vi "Application Error Class Constructor.vi"(0 "Application Error in":refnum<class "Application Error.lvclass">, 1 "Error Scope":string, 2 "Error Name":string, 5 "Error Source":string, 7 "Log Error?":bool, 9 "Call Chain":string[](array[string]), 11 "error in (no error)":errorcluster, 12 "Error Message":string, 13 "Time Stamp":timestamp) -> (15 "error out":errorcluster)   [LabVIEW 2016, in "Stream Error.lvlib" / "Application Error.lvclass"]
doc: "--\nCopyright © 2017 Composed SystemsI All rights reserved.\n\nAuthor: Jon McBee <jon.mcbee@composed.io>\n\nThis library is provided \"AS IS\" ,WITHOUT WARRANTIES OR\nCONDITIONS OF ANY KIND, either express or implied.\n\nComposed Systems -- composed.io\n\nStream 0.0.1.1\nJon McBee - Composed Systems\nCopyright (c) 2017, Composed Systems"
uses:
  <userlib>/Composed Systems/Stream/Error/Classes/Application Error/Application Error.lvclass
  C:/Program Files (x86)/National Instruments/LabVIEW 2016/user.lib/Composed Systems/Stream/Error/Classes/Error Interface/Error Interface.lvclass
  <userlib>/Composed Systems/Stream/Error/Classes/Error Interface/Error Interface.lvclass/Error Interface.ctl
  <userlib>/Composed Systems/Stream/Log/Application Log/Log Level.ctl
  <userlib>/Composed Systems/Stream/Error/Classes/Error Interface/Error Interface.lvclass
  <userlib>/Composed Systems/Stream/Log/Global Application Log/Global Application Log.lvclass
  <userlib>/Composed Systems/Stream/Log/Application Log/Application Log.lvclass
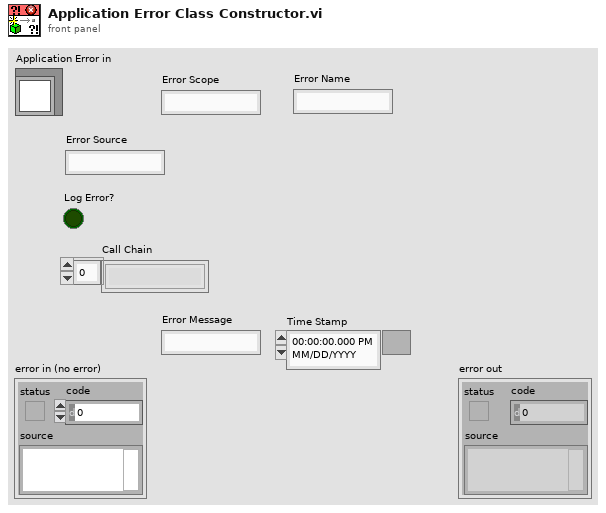
[diagram p1: front panel]
types:
  T1 = typedef "Stream Log.lvlib/Application Log.lvclass/Log Level.ctl" = enum16{"Imperative", "Major", "Minor", "Debug", "Off"}
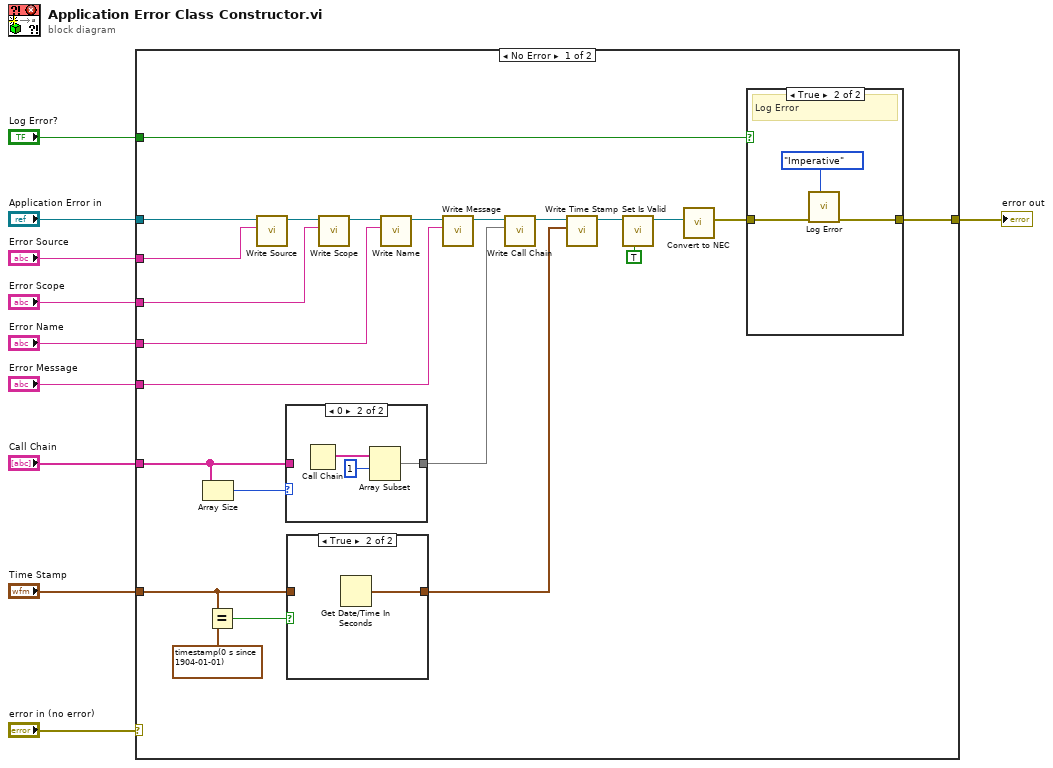
[diagram p0: block diagram]
diagram:
  n1 = case shown="No Error" "error in (no error)" {
    selector: "error in (no error)" -> [_ w44]
    tunnel: "Log Error?" -> [w14 _]
    tunnel: "Time Stamp" -> [w31 _]
    tunnel: "Call Chain" -> [w29 _]
    tunnel: "Error Source" -> [w28 _]
    tunnel: "Error Scope" -> [w27 _]
    tunnel: "Error Name" -> [w21 _]
    tunnel: "Error Message" -> [w20 _]
    tunnel: [w12 w44] -> w1
    tunnel: "Application Error in" -> [w11 _]
    frame No Error {
      n2 = Array Size(array=w29) -> (size(s)=w30:i32)
      n3 = Equal?(x=w31, y=timestamp(0 s since 1904-01-01)) -> (x = y?=w32:bool)
      n4 = call <userlib>:"Write Source.vi"("Source"=w28, "Error Interface in"=w11) -> ("Error Interface out"=w26:refnum<class "Application Error.lvclass">)  [unwired: 8 in, 1 out]
      n5 = case shown="0" w30 {
        tunnel: [w38 w39] -> w19
        tunnel: w29 -> [w38 _]
        frame Default {
        }
        frame 0 {
          n6 = Call Chain() -> (call chain=w41:string[])
          n7 = Array Subset(array=w41, index=1 ("length")) -> (w39:string[])  [unwired: 1 in]
        }
      }
      n8 = case shown="True" w32 {
        tunnel: [w42 w43] -> w18
        tunnel: w31 -> [w42 _]
        frame False {
        }
        frame True {
          n9 = Get Date/Time In Seconds() -> (seconds since 1Jan1904=w43:timestamp)
        }
      }
      n10 = call <userlib>:"Write Scope.vi"("Scope"=w27, "Error Interface in"=w26) -> ("Error Interface out"=w25:refnum<class "Application Error.lvclass">)  [unwired: 8 in, 1 out]
      n11 = call <userlib>:"Write Name.vi"("Name"=w21, "Error Interface in"=w25) -> ("Error Interface out"=w24:refnum<class "Application Error.lvclass">)  [unwired: 8 in, 1 out]
      n12 = call <userlib>:"Write Message.vi"("Message"=w20, "Error Interface in"=w24) -> ("Error Interface out"=w23:refnum<class "Application Error.lvclass">)  [unwired: 8 in, 1 out]
      n13 = call <userlib>:"Write Call Chain.vi"("Call Chain"=w19, "Error Interface in"=w23) -> ("Error Interface out"=w22:refnum<class "Application Error.lvclass">)  [unwired: 8 in, 1 out]
      n14 = call <userlib>:"Write Time Stamp.vi"("Time Stamp"=w18, "Error Interface in"=w22) -> ("Error Interface out"=w17:refnum<class "Application Error.lvclass">)  [unwired: 8 in, 1 out]
      n15 = call <userlib>:"Set Is Valid.vi"("Valid"=TRUE, "Error Interface in"=w17) -> ("Error Interface out"=w15:refnum<class "Application Error.lvclass">)  [unwired: 9 in]
      n16 = call <userlib>:"Convert to NEC.vi"("Error Interface in"=w15) -> ("error out"=w13:errorcluster)  [unwired: 10 in]
      n17 = case shown="True" w14 {
        tunnel: w13 -> [w34 w37]
        tunnel: [w34 w36] -> w12
        frame False {
          # "Dont Log Error"
        }
        frame True {
          # "Log Error"
          n18 = call <userlib>:"Log Error.vi"("Level"=Log_Level."Imperative", "error in (no error)"=w37) -> ("error out"=w36:errorcluster)  [unwired: 9 in]
        }
      }
    }
    frame Error {
    }
  }
  "error out" <- w1
